vi "CSTK_Icon_Creator_Insert.vi"(0 "字符":string, 1 "模板选择":T1, 3 "LOGO":string, 5 "字体颜色":u32(colorbox), 7 "字体":enum16{"Small Fonts", "6px2bus"}(ring), 9 "水平偏移":i8, 11 "error in (no error)":errorcluster caption="错误输入（无错误）", 12 "标题背景色":u32(colorbox)=16777215, 14 "主体背景色":u32(colorbox)=16777215) -> (4 "图片":picture, 6 "图片数据":T2 caption="图像数据", 15 "error out":errorcluster caption="错误输出")   [LabVIEW 2015, in "CSTK_Icon Creator.lvlib"]
uses:
  CSTK_Icon Creator.lvlib
  <vilib>/picture/picture.llb/imagedata.ctl
  CSTK_Icon_Creator_Template.ctl
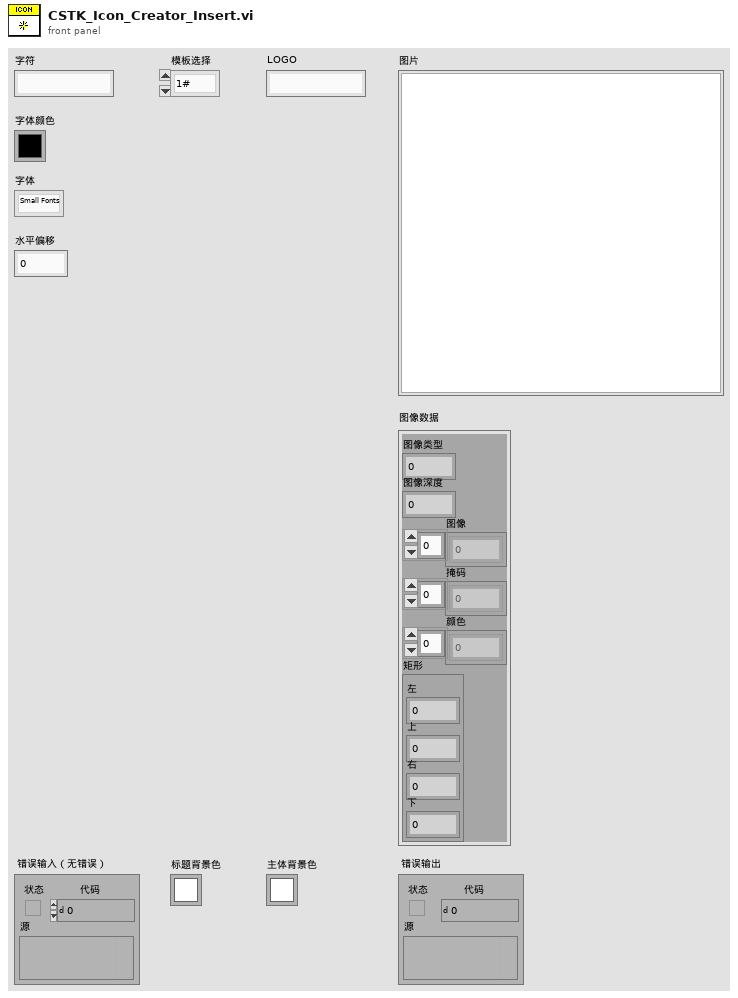
[diagram p1: front panel]
types:
  T1 = typedef "CSTK_Icon Creator.lvlib/CSTK_Icon_Creator_Template.ctl" = enum16{"1#", "2#", "3#", "4#", "Ctl"}
  T2 = typedef "imagedata.ctl" = cluster{"image type":i32, "image depth":i32, "image":u8[], "mask":u8[], "colors":u32[], "Rectangle":cluster{"left":i16, "top":i16, "right":i16, "bottom":i16}}
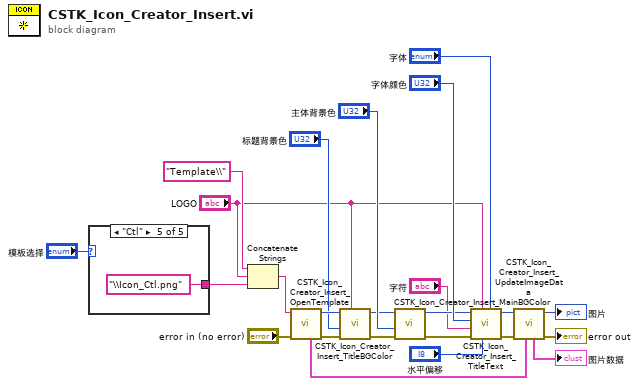
[diagram p0: block diagram]
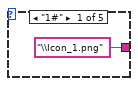
[diagram p2: hidden frame]
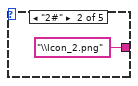
[diagram p3: hidden frame]
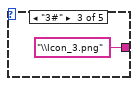
[diagram p4: hidden frame]
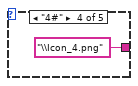
[diagram p5: hidden frame]
diagram:
  n1 = case shown="\"Ctl\"" "模板选择" {
    tunnel: ["\\Icon_1.png" ("名称或相对路径") "\\Icon_2.png" ("名称或相对路径") "\\Icon_3.png" ("名称或相对路径") "\\Icon_4.png" ("名称或相对路径") "\\Icon_Ctl.png" ("名称或相对路径")] -> w3
    frame "1#" {
    }
    frame "2#" {
    }
    frame "3#" {
    }
    frame "4#" {
    }
    frame "Ctl" {
    }
  }
  n2 = Concatenate Strings("Template\\" ("字符串"), "LOGO", w3) -> (w2:string)
  n3 = call "CSTK_Icon_Creator_Insert_OpenTemplate.vi"("错误输入（无错误）"="error in (no error)", "模板相对路径"=w2) -> ("错误输出"=w19:errorcluster, "图片输出"=w21:picture, "图片数据输出"=w8:T2)  [unwired: 7 in]
  n4 = call "CSTK_Icon_Creator_Insert_TitleBGColor.vi"("LOGO"="LOGO", "error in (no error)"=w19, "标题背景色"="标题背景色", "图片输入"=w21) -> ("error out"=w16:errorcluster, "图片输出"=w17:picture)  [unwired: 6 in]
  n5 = call "CSTK_Icon_Creator_Insert_MainBGColor.vi"("error in (no error)"=w16, "主体背景色"="主体背景色", "图片输入"=w17) -> ("error out"=w13:errorcluster, "图片输出"=w15:picture)  [unwired: 7 in]
  n6 = call "CSTK_Icon_Creator_Insert_TitleText.vi"("字体"="字体", "水平偏移"="水平偏移", "LOGO"="LOGO", "error in (no error)"=w13, "字符"="字符", "字体颜色"="字体颜色", "图片输入"=w15) -> ("error out"=w10:errorcluster, "图片输出"=w11:picture)  [unwired: 3 in]
  n7 = call "CSTK_Icon_Creator_Insert_UpdateImageData.vi"("图片数据输入"=w8, "error in (no error)"=w10, "图片输入"=w11) -> ("error out"=→"error out":errorcluster, "图片输出"=→"图片":picture, "图片数据输出"=→"图片数据":T2)  [unwired: 6 in]
